vi "_Read No Objects - Power Meter.vi"(5 "VISA Resource Name Out":refnum<visa-resource-name>, 8 "error in (no error)":errorcluster, 10 "VISA Resource Name In":refnum<visa-resource-name>, 11 "Power Meter in":T1={"Wavelength"=0.0, "AVG"=0, "Range"=0, "Backlight"=0, "Beeper"=0, "Zero"=0, "Local Lockout"=0, "ATTN"=0, "Run/Stop"=0, "Units"=0, "Averaging Time"=0.0, "Averaging"=TRUE, "Most Recent Power"=0.0, "Filter"=0}) -> (0 "error out":errorcluster, 2 "X array":dbl[](array[numeric]), 3 "Power Meter Out":T1={"Wavelength"=0.0, "AVG"=0, "Range"=0, "Backlight"=0, "Beeper"=0, "Zero"=0, "Local Lockout"=0, "ATTN"=0, "Run/Stop"=0, "Units"=0, "Averaging Time"=0.0, "Averaging"=TRUE, "Most Recent Power"=0.0, "Filter"=0})   [LabVIEW 2012]
doc: "(Protected, Dynamic, Pure Virtual/Abstract) Perform a measurement and return one or more channels of data. Outsiders should not call this method, but instead the public \"Read Power.vi\".\n\nThis vi compares the current point to the previous and returns 0 if current if more than twice as much as previous. It also creates a warning, error value of 1."
uses:
  Newport 1830-C/Newport 1830-C.lvlib
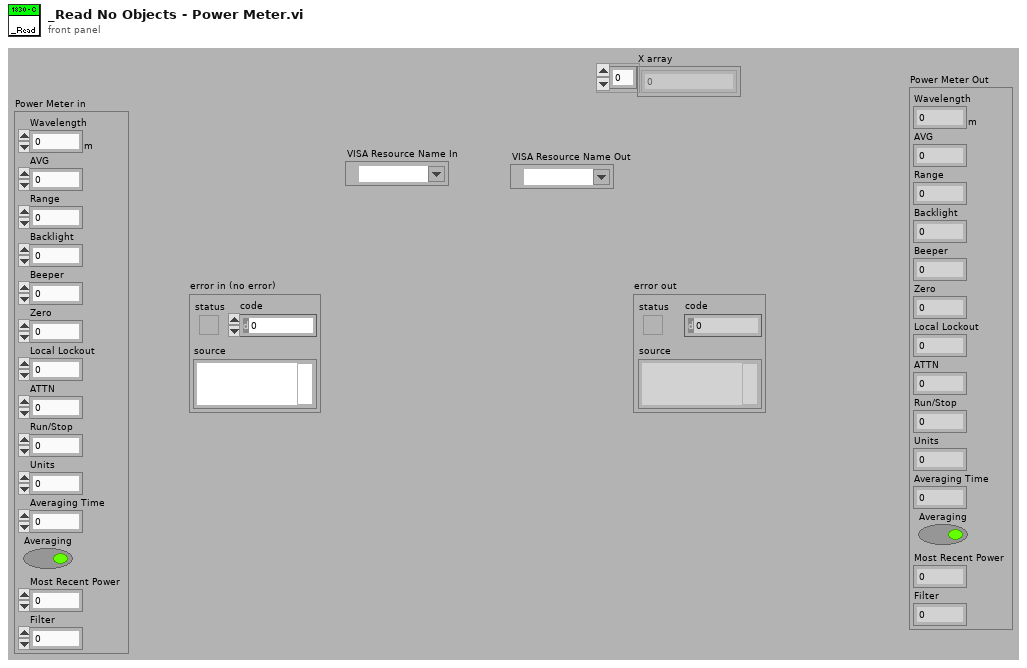
[diagram p1: front panel]
types:
  T1 = cluster{"Wavelength":dbl[unit], "AVG":i32, "Range":i32, "Backlight":i32, "Beeper":i32, "Zero":i32, "Local Lockout":i32, "ATTN":i32, "Run/Stop":i32, "Units":i32, "Averaging Time":dbl, "Averaging":bool, "Most Recent Power":dbl, "Filter":i32}
  T2 = typedef "Filters.ctl" = u16
  T3 = cluster{"Wavelength":dbl[unit], "AVG":u16, "Range":u16, "Backlight":u16, "Beeper":u16, "Zero":u16, "Local Lockout":u16, "ATTN":u16, "Run/Stop":u16, "Units":u16, "Averaging Time":dbl, "Averaging":bool, "Most Recent Power":dbl, "Filter":T2}
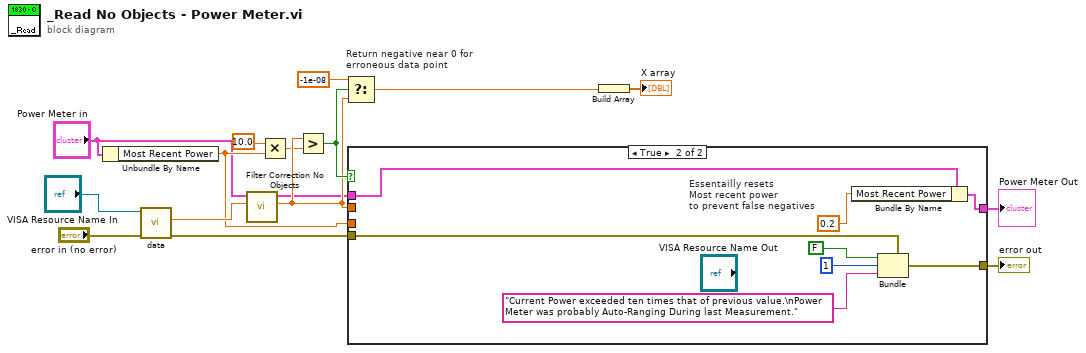
[diagram p0: block diagram]
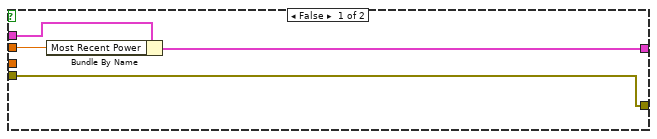
[diagram p2: hidden frame]
diagram:
  n1 = Unbundle By Name("Power Meter in") -> ("Most Recent Power"=w7:dbl)
  n2 = call "data.vi"("error in (no error)"="error in (no error)", "VISA resource name"="VISA Resource Name In") -> ("error out"=w4:errorcluster, "Power"=w11:dbl)  [unwired: 7 in, 1 out]
  n3 = call "Filter Correction No Objects.vi"("Read Power"=w11, "Cluster In"="Power Meter in") -> ("Corrected Power"=w10:dbl, "Cluster Out"=w3:T3)  [unwired: 8 in]
  n4 = Multiply(x=10.0, y=w7) -> (x*y=w8:dbl)
  n5 = Greater?(x=w10, y=w8) -> (0:w14:bool)
  n6 = Select "Return negative near 0 for\nerroneous data point"(t=-1e-08, s=w14, f=w10) -> (s? t:f=w12:dbl)
  n7 = case shown="True" w14 {
    tunnel: w4 -> [w20 w28]
    tunnel: [w20 w24] -> w13
    tunnel: w3 -> [w19 w23]
    tunnel: w10 -> [w17 _]
    tunnel: [w18 w22] -> w2
    tunnel: w7 -> [_ _]
    frame False {
      n8 = Bundle By Name(cluster=w19, "Most Recent Power"=w17) -> (w18:T3)
    }
    frame True {
      w21 = 0.2  # Essentailly resets Most recent power to prevent false negatives
      n9 = Bundle By Name(cluster=w23, "Most Recent Power"=w21) -> (w22:T3)
      n10 = Bundle(cluster=w28, "status"=FALSE, "code"=1, "source"="Current Power exceeded ten times that of previous value.\nPower Meter was probably Auto-Ranging During last Measurement.") -> (w24:errorcluster)
    }
  }
  "error out" <- w13
  "Power Meter Out" <- w2
  n11 = Build Array(w12) -> (→"X array":dbl[])
